vi "NeuronID_UDP_send_v003.vi"(2 "error in (no error)":errorcluster, 3 "Neuron ID":dbl(slide) scale=0.0..10.0, 4 "Address selector":i32[](array[numeric]), 5 "UDP Network Connection in":refnum<k16>) -> (0 "error out":errorcluster, 1 "UDP Network Connection out":refnum<k16>)   [LabVIEW 2019]
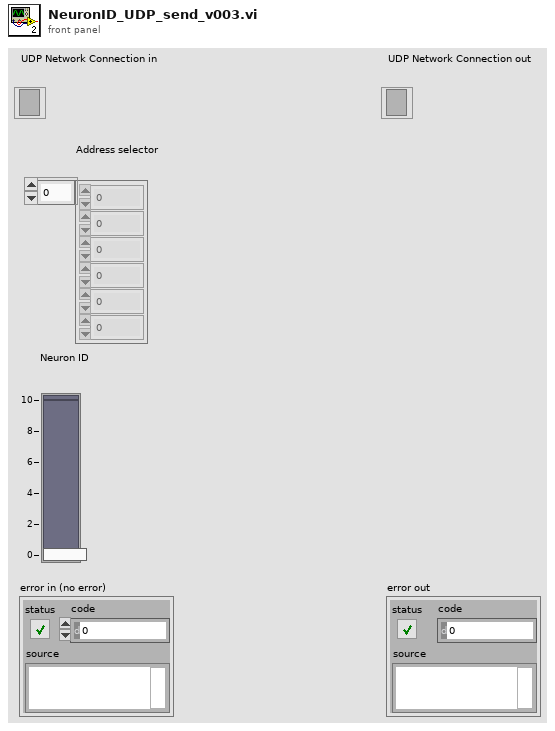
[diagram p1: front panel]
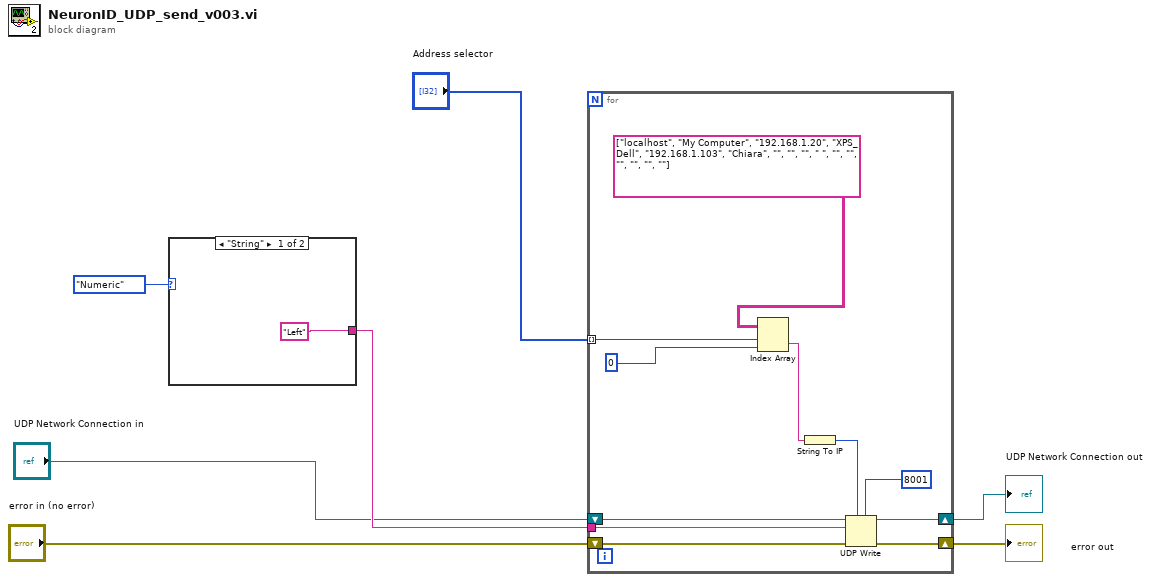
[diagram p0: block diagram]
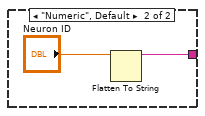
[diagram p2: hidden frame]
diagram:
  n1 = case shown="\"String\"" enum16{"String", "Numeric"}."Numeric" ("Data to send") {
    tunnel: ["Left" ("Message") w9] -> w6
    frame "String" {
    }
    frame "Numeric", Default {
      n2 = Flatten To String(anything="Neuron ID") -> (data string=w9:string)  [unwired: 3 in, 2 out]
    }
  }
  n3 = for {
    tunnel: w6 -> [w15]
    shift-right: [w20] -> w2
    shift-left: "error in (no error)" -> [w21]
    shift-right: [w18] -> w4
    shift-left: "UDP Network Connection in" -> [w19]
    tunnel: "Address selector" -> [w12] mode=indexing
    n4 = Index Array(array=string[][] [["localhost", "My Computer"], ["192.168.1.20", "XPS_Dell"], ["192.168.1.103", "Chiara"], ["", ""], ["", " "], ["", ""], ["", ""], ["", ""]] ("Address list"), index (row)=w12, index (col)=0 ("disabled index (col)")) -> (element=w13:string)
    n5 = String To IP(1:w13) -> (0:w16:u32)
    n6 = UDP Write(address=w16, port or service name=u16 8001, connection ID=w19, data in=w15, 8:w21) -> (error out=w20:errorcluster, 3:w18:refnum<k16>)  [unwired: 1 in]
  }
  "UDP Network Connection out" <- w4
  "error out" <- w2
